vi "TxRS232.vi"(0 "VISA resource name":refnum<visa-resource-name>="COM5", 1 "Data":string) -> ()   [LabVIEW 2014]
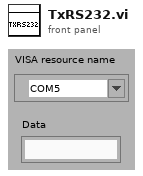
[diagram p1: front panel]
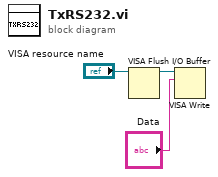
[diagram p0: block diagram]
diagram:
  n1 = VISA Flush I/O Buffer(VISA resource name="VISA resource name") -> (VISA resource name out=w1:refnum<visa-resource-name>)  [unwired: 2 in, 1 out]
  n2 = VISA Write(VISA resource name=w1, write buffer="Data") -> ()  [unwired: 1 in, 3 out]
